vi "mod_query.vi"(5 "connection reference":T3) -> ()   [LabVIEW 2018]
uses:
  <vilib>/addons/database/Connection.llb/Conn ObjectReference.ctl
  <vilib>/addons/database/Connection.llb/Conn Execute.vi
  <vilib>/addons/database/Recordset.llb/Rec Fetch Recordset Data (R).vi
  <vilib>/addons/database/_DB Variant To Data/Database Variant To Data.xnode
  <vilib>/addons/database/NI_Database_API.lvlib
panel:
  in  "清除指示灯 2":bool
  in  "查询学生":bool
  in  "学生信息输入框":T1
  out "数值":dbl
  in  "信息框":i32(listbox)
  in  "查询宿舍所住人信息":bool
  in  "清除指示灯":bool
  in  "查询按钮":bool
  in  "信息输入框":T2
  in  "刷新按钮":bool
  in  "已编辑行数组":u32[](array[numeric])
  in  "信息框缓冲备份":string[][](array[string])
  in  "error in (no error)":errorcluster
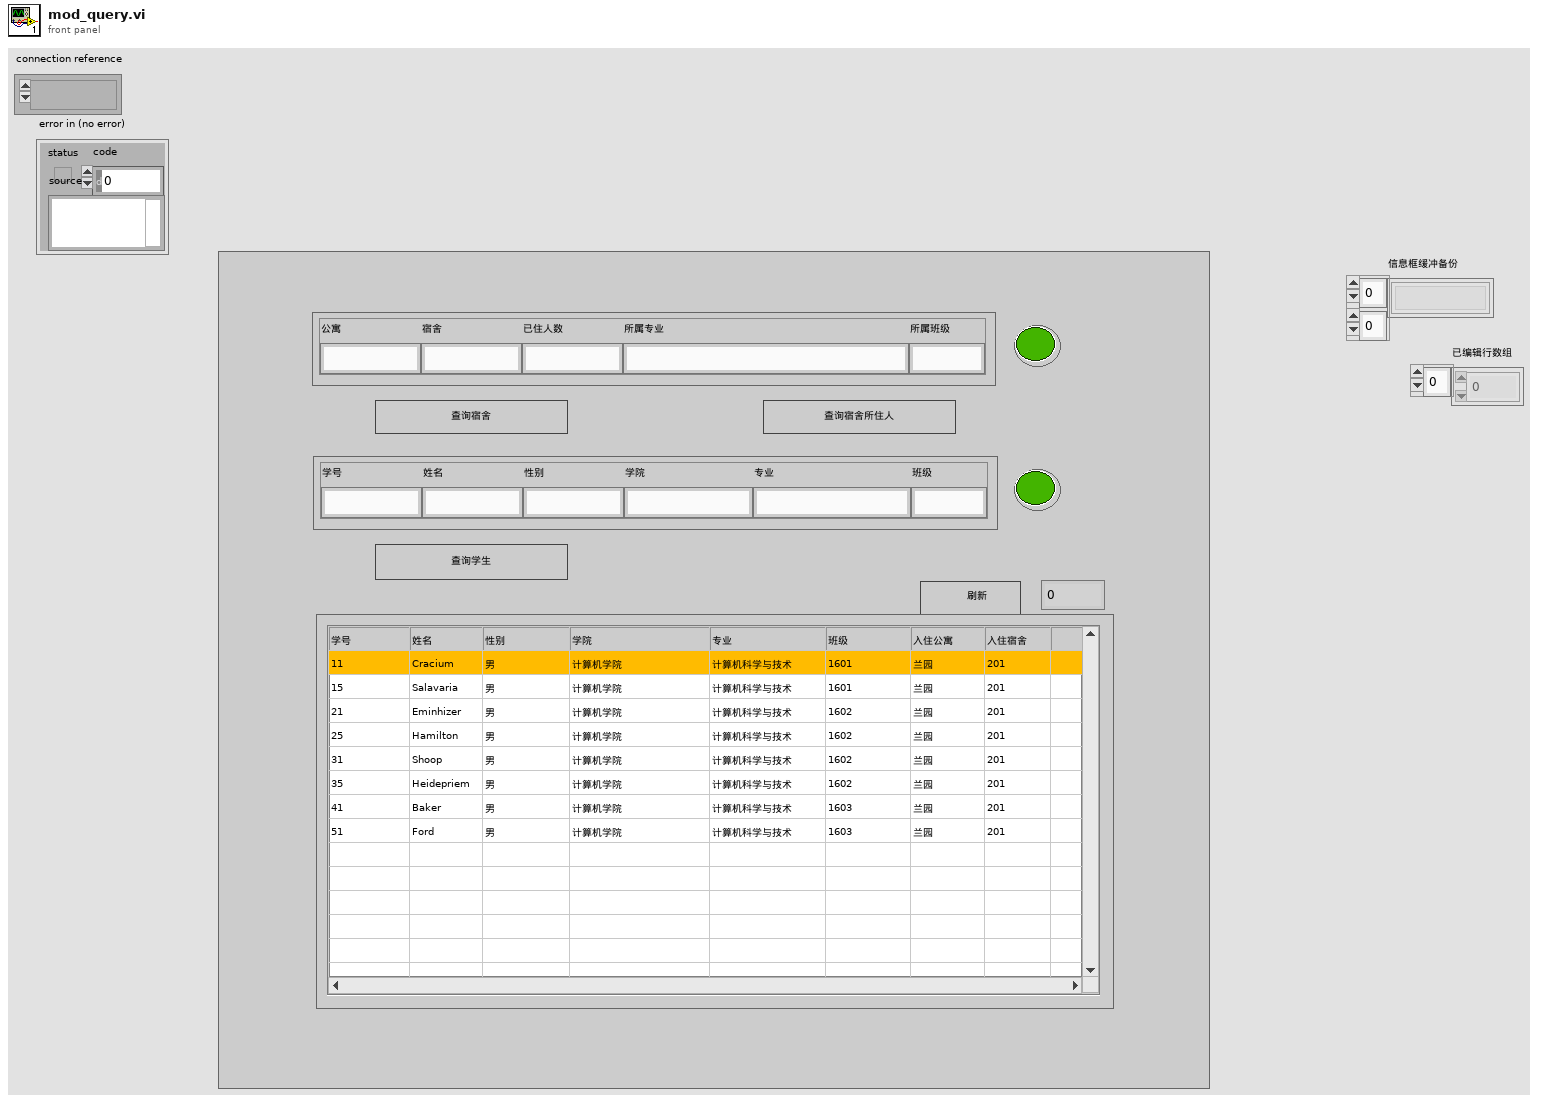
[diagram p1: front panel]
types:
  T1 = cluster{"学号":string, "姓名":string, "性别":string, "学院":string, "专业":string, "班级":string}
  T2 = cluster{"公寓":string, "宿舍":string, "已住人数":string, "所属专业":string, "所属班级":string}
  T3 = typedef "NI_Database_API.lvlib/Conn ObjectReference.ctl" = refnum<k1>
  T4 = cluster{string, string, string, string, string, string, string, string}
  T5 = cluster{string, string, string, string, string, string}
  T6 = typedef "NI_Database_API.lvlib/Rec ObjectReference.ctl" = refnum<k1>
  T7 = cluster{string, string, string, string, string}[]
  T8 = cluster{string, string, string, string, string, string, string, string}[]
  T9 = cluster{string, string, string, string, string, string}[]
  T10 = cluster{"[0]":string, "[1]":string, "[2]":string, "[3]":string, "[4]":string}
  T11 = cluster{"[0]":string, "[1]":string, "[2]":string, "[3]":string, "[4]":string, "[5]":string}
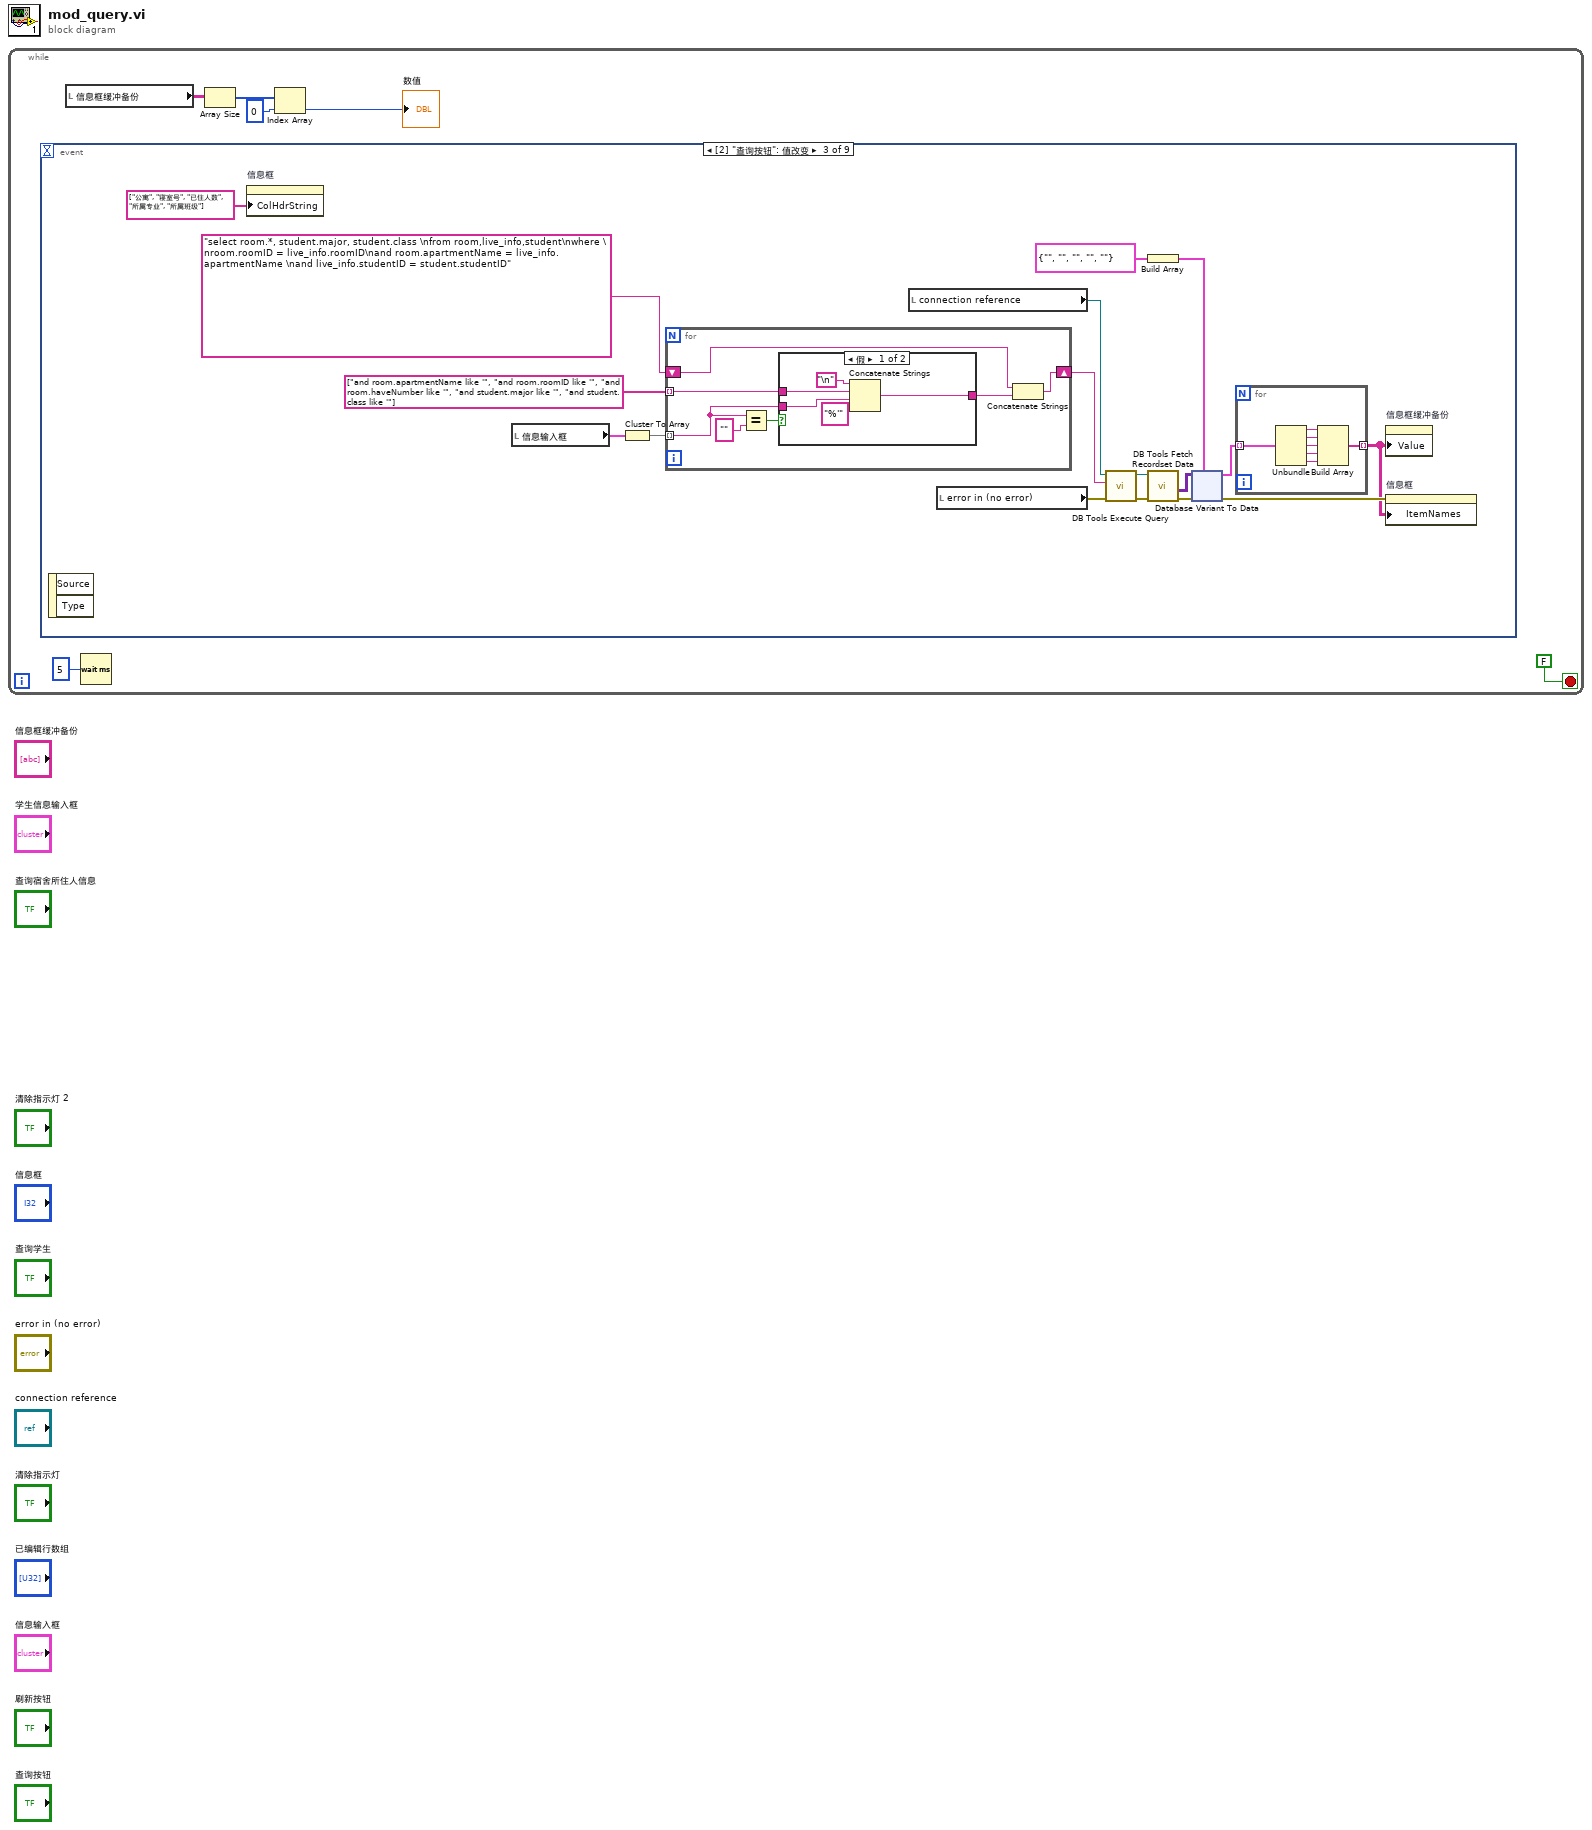
[diagram p0: block diagram]
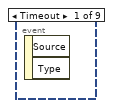
[diagram p2: hidden frame]
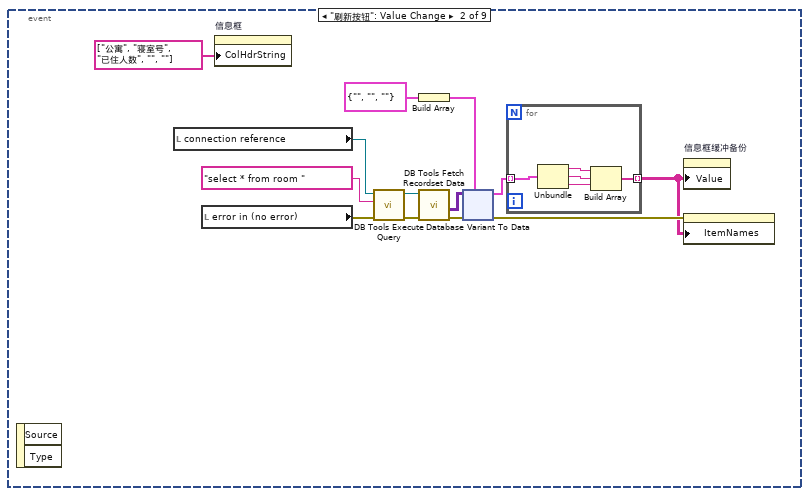
[diagram p3: hidden frame]
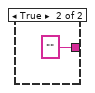
[diagram p4: hidden frame]
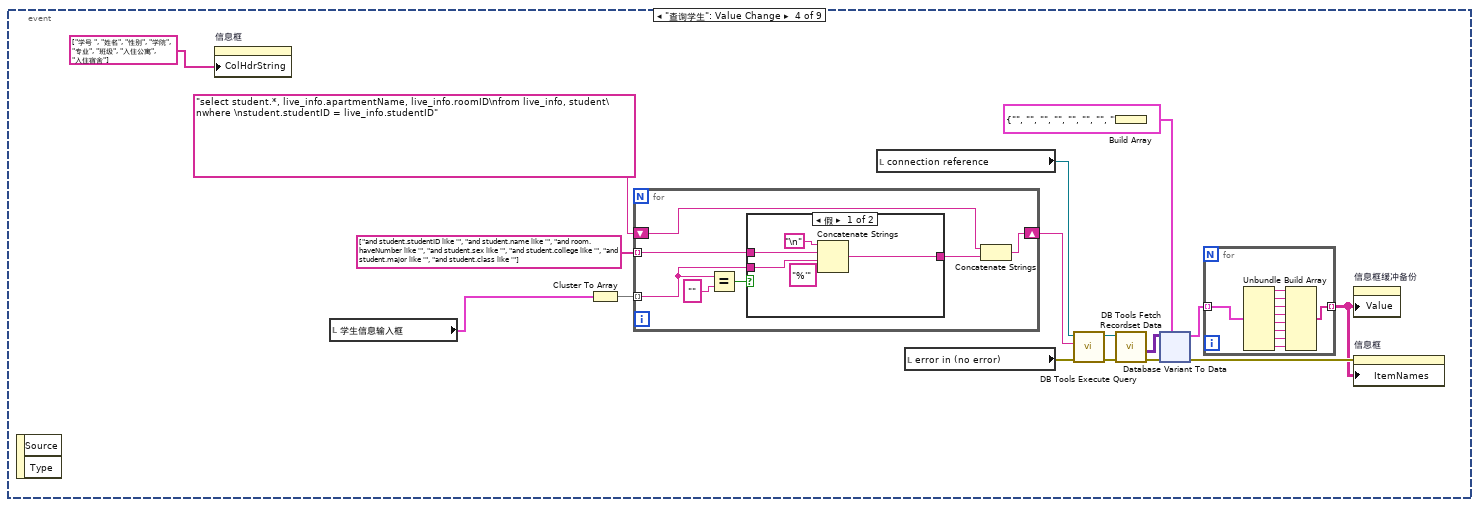
[diagram p5: hidden frame]
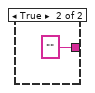
[diagram p6: hidden frame]
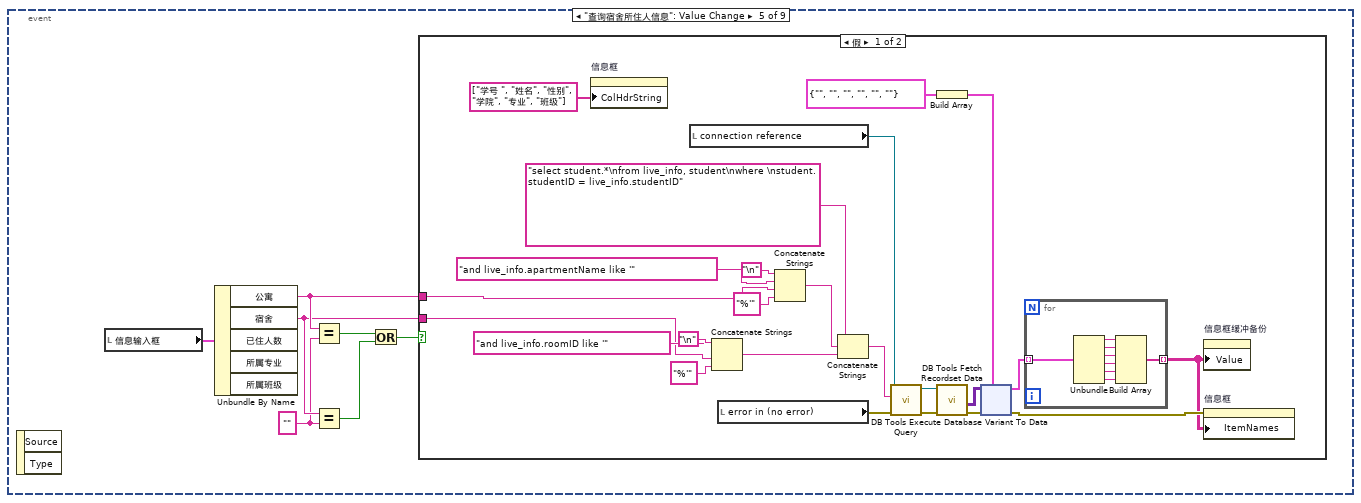
[diagram p7: hidden frame]
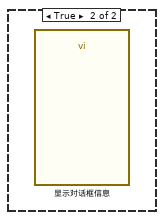
[diagram p8: hidden frame]
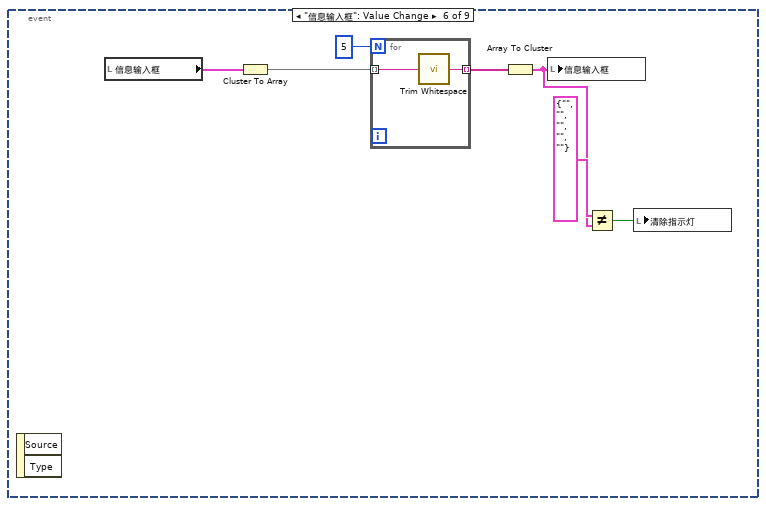
[diagram p9: hidden frame]
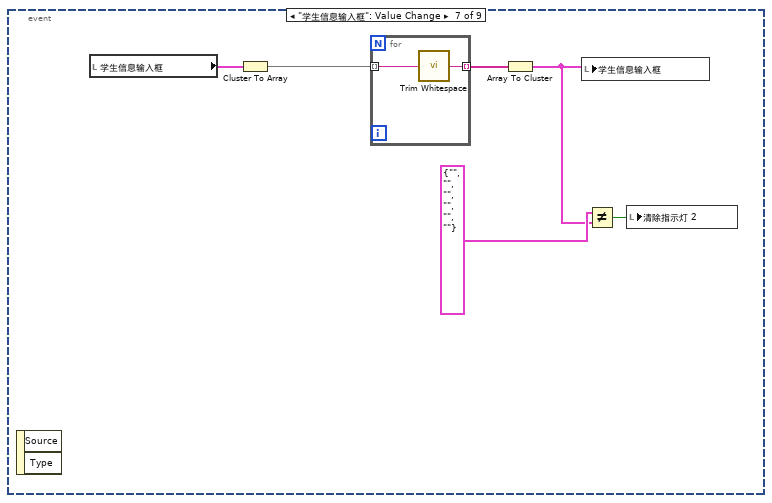
[diagram p10: hidden frame]
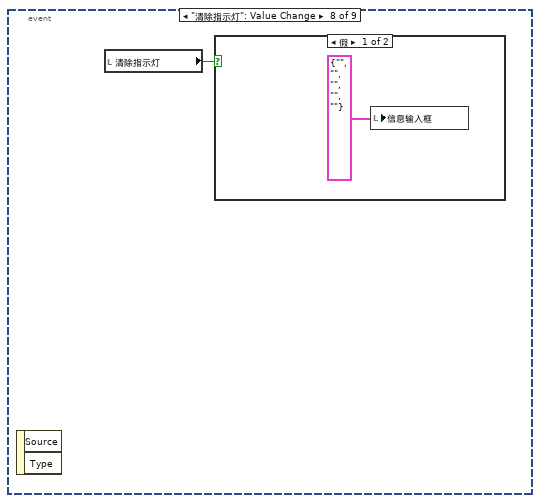
[diagram p11: hidden frame]
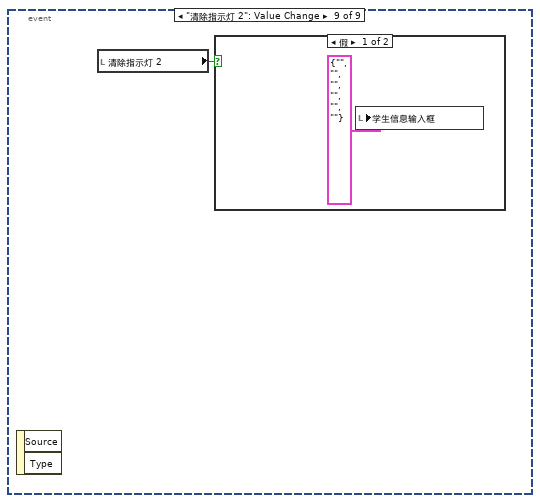
[diagram p13: hidden frame]
diagram:
  n1 = while {
    stop <- FALSE stop-if-true
    n2 = event shown="[2] \"查询按钮\": 值改变" {
      selector: _ -> [_ _ _ _ _ _ _ _ _]
      dyn-events: _ -> [_ _ _ _ _ _ _ _ _]
      timeout: _ -> [_ _ _ _ _ _ _ _ _]
      event Timeout {
        n3 = event-data() -> ()  [unwired: 1 in, 2 out]
      }
      event "刷新按钮": Value Change {
        n4 = event-data() -> ()  [unwired: 1 in, 2 out]
        n5 = local read "connection reference"() -> (w13:T3)
        n6 = local read "error in (no error)"() -> (w12:errorcluster)
        n7 = property on="信息框" class="MCListbox (严格)"("ColHdrString"=string[] ["公寓", "寝室号", "已住人数", "", ""] ("列首字符串[]")) -> ()  [unwired: 2 in, 2 out]
        n8 = call-poly <vilib>:"DB Tools Execute Query.vi"("error in (no error)"=w12, "SQL query"="select * from room ", "connection reference"=w13) -> ("error out"=w15:errorcluster, "recordset reference"=w14:T6)  [unwired: 5 in]
        n9 = Build Array(cluster{string, string, string} {"", "", ""}) -> (w17:cluster{string, string, string}[])
        n10 = call-poly <vilib>:"DB Tools Fetch Recordset Data.vi"("error in (no error)"=w15, "recordset reference"=w14) -> ("error out"=w16:errorcluster, "recordset data"=w11:variant[][])  [unwired: 3 in, 1 out]
        n11 = xnode "Database Variant To Data"("database variant"=w11, "error in (no error)"=w16, "type"=w17) -> ("data"=w18:cluster{string, string, string}[], "error out"=w19:errorcluster)
        n12 = for {
          tunnel: w18 -> [w23] mode=indexing
          tunnel: [w24] -> w8 mode=indexing
          n13 = Unbundle(w23) -> (w21:string, w22:string, w20:string)
          n14 = Build Array(w21, w22, w20) -> (w24:string[])
        }
        n15 = property on="信息框缓冲备份" class="Arr (严格)"("Value"=w8) -> ()  [unwired: 2 in, 2 out]
        n16 = property on="信息框" class="MCListbox (严格)"(error in=w19, "ItemNames"=w8) -> ()  [unwired: 1 in, 2 out]
      }
      event "查询按钮": Value Change {
        n17 = event-data() -> ()  [unwired: 1 in, 2 out]
        n18 = property on="信息框" class="MCListbox (严格)"("ColHdrString"=string[] ["公寓", "寝室号", "已住人数", "所属专业", "所属班级"] ("列首字符串[]")) -> ()  [unwired: 2 in, 2 out]
        n19 = local read "信息输入框"() -> (w134:T2)
        n20 = Cluster To Array(cluster=w134) -> (array=w133:string[])
        n21 = for {
          shift-right: [w147] -> w135
          shift-left: "select room.*, student.major, student.class \nfrom room,live_info,student\nwhere \nroom.roomID = live_info.roomID\nand room.apartmentName = live_info.apartmentName \nand live_info.studentID = student.studentID" -> [w146]
          tunnel: string[] ["and room.apartmentName like '", "and room.roomID like '", "and room.haveNumber like '", "and student.major like '", "and student.class like '"] ("数组") -> [w148] mode=indexing
          tunnel: w133 -> [w149] mode=indexing
          n22 = Equal?(x=w149, y="") -> (x = y?=w151:bool)
          n23 = case shown="假" w151 {
            tunnel: [w152 ""] -> w145
            tunnel: w149 -> [w154 _]
            tunnel: w148 -> [w155 _]
            frame False {
              n24 = Concatenate Strings("\n", w155, w154, "%'") -> (w152:string)
            }
            frame True {
            }
          }
          n25 = Concatenate Strings(w146, w145) -> (w147:string)
        }
        n26 = local read "connection reference"() -> (w144:T3)
        n27 = local read "error in (no error)"() -> (w143:errorcluster)
        n28 = call-poly <vilib>:"DB Tools Execute Query.vi"("error in (no error)"=w143, "SQL query"=w135, "connection reference"=w144) -> ("error out"=w136:errorcluster, "recordset reference"=w137:T6)  [unwired: 5 in]
        n29 = Build Array(cluster{string, string, string, string, string} {"", "", "", "", ""}) -> (w140:T7)
        n30 = call-poly <vilib>:"DB Tools Fetch Recordset Data.vi"("error in (no error)"=w136, "recordset reference"=w137) -> ("error out"=w138:errorcluster, "recordset data"=w139:variant[][])  [unwired: 3 in, 1 out]
        n31 = xnode "Database Variant To Data"("database variant"=w139, "error in (no error)"=w138, "type"=w140) -> ("data"=w141:T7, "error out"=w142:errorcluster)
        n32 = for {
          tunnel: w141 -> [w163] mode=indexing
          tunnel: [w164] -> w128 mode=indexing
          n33 = Unbundle(w163) -> (w162:string, w161:string, w160:string, w159:string, w158:string)
          n34 = Build Array(w162, w161, w160, w159, w158) -> (w164:string[])
        }
        n35 = property on="信息框缓冲备份" class="Arr (严格)"("Value"=w128) -> ()  [unwired: 2 in, 2 out]
        n36 = property on="信息框" class="MCListbox (严格)"(error in=w142, "ItemNames"=w128) -> ()  [unwired: 1 in, 2 out]
      }
      event "查询学生": Value Change {
        n37 = event-data() -> ()  [unwired: 1 in, 2 out]
        n38 = property on="信息框" class="MCListbox (严格)"("ColHdrString"=string[] ["学号 ", "姓名", "性别", "学院", "专业", "班级", "入住公寓", "入住宿舍"] ("列首字符串[]")) -> ()  [unwired: 2 in, 2 out]
        n39 = local read "学生信息输入框"() -> (w330:T1)
        n40 = Cluster To Array(cluster=w330) -> (array=w336:string[])
        n41 = for {
          shift-right: [w349] -> w337
          shift-left: "select student.*, live_info.apartmentName, live_info.roomID\nfrom live_info, student\nwhere \nstudent.studentID = live_info.studentID" -> [w348]
          tunnel: string[] ["and student.studentID like '", "and student.name like '", "and room.haveNumber like '", "and student.sex like '", "and student.college like '", "and student.major like '", "and student.class like '"] ("数组") -> [w350] mode=indexing
          tunnel: w336 -> [w351] mode=indexing
          n42 = Equal?(x=w351, y="") -> (x = y?=w353:bool)
          n43 = case shown="假" w353 {
            tunnel: [w354 ""] -> w347
            tunnel: w351 -> [w356 _]
            tunnel: w350 -> [w357 _]
            frame False {
              n44 = Concatenate Strings("\n", w357, w356, "%'") -> (w354:string)
            }
            frame True {
            }
          }
          n45 = Concatenate Strings(w348, w347) -> (w349:string)
        }
        n46 = local read "connection reference"() -> (w346:T3)
        n47 = local read "error in (no error)"() -> (w345:errorcluster)
        n48 = call-poly <vilib>:"DB Tools Execute Query.vi"("error in (no error)"=w345, "SQL query"=w337, "connection reference"=w346) -> ("error out"=w338:errorcluster, "recordset reference"=w339:T6)  [unwired: 5 in]
        n49 = Build Array(T4 {"", "", "", "", "", "", "", ""}) -> (w342:T8)
        n50 = call-poly <vilib>:"DB Tools Fetch Recordset Data.vi"("error in (no error)"=w338, "recordset reference"=w339) -> ("error out"=w340:errorcluster, "recordset data"=w341:variant[][])  [unwired: 3 in, 1 out]
        n51 = xnode "Database Variant To Data"("database variant"=w341, "error in (no error)"=w340, "type"=w342) -> ("data"=w343:T8, "error out"=w344:errorcluster)
        n52 = for {
          tunnel: w343 -> [w368] mode=indexing
          tunnel: [w369] -> w332 mode=indexing
          n53 = Unbundle(w368) -> (w367:string, w366:string, w365:string, w364:string, w363:string, w360:string, w361:string, w362:string)
          n54 = Build Array(w367, w366, w365, w364, w363, w360, w361, w362) -> (w369:string[])
        }
        n55 = property on="信息框缓冲备份" class="Arr (严格)"("Value"=w332) -> ()  [unwired: 2 in, 2 out]
        n56 = property on="信息框" class="MCListbox (严格)"(error in=w344, "ItemNames"=w332) -> ()  [unwired: 1 in, 2 out]
      }
      event "查询宿舍所住人信息": Value Change {
        w628 = ""
        n57 = event-data() -> ()  [unwired: 1 in, 2 out]
        n58 = local read "信息输入框"() -> (w634:T2)
        n59 = Unbundle By Name(w634) -> ("公寓"=w633:string, "宿舍"=w629:string)  [unwired: 3 out]
        n60 = Equal?(x=w633, y=w628) -> (x = y?=w631:bool)
        n61 = Equal?(x=w629, y=w628) -> (x = y?=w630:bool)
        n62 = Or(x=w631, y=w630) -> (x .or. y?=w632:bool)
        n63 = case shown="假" w632 {
          tunnel: w633 -> [w643 _]
          tunnel: w629 -> [w635 _]
          frame False {
            n64 = property on="信息框" class="MCListbox (严格)"("ColHdrString"=string[] ["学号 ", "姓名", "性别", "学院", "专业", "班级"] ("列首字符串[]")) -> ()  [unwired: 2 in, 2 out]
            n65 = local read "connection reference"() -> (w658:T3)
            n66 = Concatenate Strings("\n", "and live_info.roomID like '" ("字符串"), w635, "%'" ("字符串")) -> (w639:string)
            n67 = local read "error in (no error)"() -> (w657:errorcluster)
            n68 = Concatenate Strings("\n", "and live_info.apartmentName like '" ("字符串"), w643, "%'" ("字符串")) -> (w640:string)
            n69 = Concatenate Strings("select student.*\nfrom live_info, student\nwhere \nstudent.studentID = live_info.studentID", w640, w639) -> (w646:string)
            n70 = call-poly <vilib>:"DB Tools Execute Query.vi"("error in (no error)"=w657, "SQL query"=w646, "connection reference"=w658) -> ("error out"=w650:errorcluster, "recordset reference"=w651:T6)  [unwired: 5 in]
            n71 = Build Array(T5 {"", "", "", "", "", ""}) -> (w654:T9)
            n72 = call-poly <vilib>:"DB Tools Fetch Recordset Data.vi"("error in (no error)"=w650, "recordset reference"=w651) -> ("error out"=w652:errorcluster, "recordset data"=w653:variant[][])  [unwired: 3 in, 1 out]
            n73 = xnode "Database Variant To Data"("database variant"=w653, "error in (no error)"=w652, "type"=w654) -> ("data"=w655:T9, "error out"=w656:errorcluster)
            n74 = for {
              tunnel: w655 -> [w665] mode=indexing
              tunnel: [w666] -> w648 mode=indexing
              n75 = Unbundle(w665) -> (w664:string, w663:string, w662:string, w661:string, w660:string, w659:string)
              n76 = Build Array(w664, w663, w662, w661, w660, w659) -> (w666:string[])
            }
            n77 = property on="信息框缓冲备份" class="Arr (严格)"("Value"=w648) -> ()  [unwired: 2 in, 2 out]
            n78 = property on="信息框" class="MCListbox (严格)"(error in=w656, "ItemNames"=w648) -> ()  [unwired: 1 in, 2 out]
          }
          frame True {
            n79 = call "显示对话框信息"() -> ()  [unwired: 10 in, 2 out]
          }
        }
      }
      event "信息输入框": Value Change {
        n80 = event-data() -> ()  [unwired: 1 in, 2 out]
        n81 = local read "信息输入框"() -> (w868:T2)
        n82 = Cluster To Array(cluster=w868) -> (array=w867:string[])
        n83 = for {
          N: 5 -> [_]
          tunnel: w867 -> [w871] mode=indexing
          tunnel: [w870] -> w869 mode=indexing
          n84 = call <vilib>:"Trim Whitespace.vi"("string"=w871) -> ("trimmed string"=w870:string)  [unwired: 1 in]
        }
        n85 = Array To Cluster(array=w869) -> (cluster=w863:T10)
        n86 = local write "信息输入框"(w863) -> ()
        n87 = Not Equal?(x=cluster{string, string, string, string, string} {"", "", "", "", ""}, y=w863) -> (x != y?=w865:bool)
        n88 = local write "清除指示灯"(w865) -> ()
      }
      event "学生信息输入框": Value Change {
        n89 = event-data() -> ()  [unwired: 1 in, 2 out]
        n90 = local read "学生信息输入框"() -> (w876:T1)
        n91 = Cluster To Array(cluster=w876) -> (array=w875:string[])
        n92 = for {
          tunnel: w875 -> [w879] mode=indexing
          tunnel: [w878] -> w877 mode=indexing
          n93 = call <vilib>:"Trim Whitespace.vi"("string"=w879) -> ("trimmed string"=w878:string)  [unwired: 1 in]
        }
        n94 = Array To Cluster(array=w877) -> (cluster=w872:T11)
        n95 = local write "学生信息输入框"(w872) -> ()
        n96 = Not Equal?(x=T5 {"", "", "", "", "", ""}, y=w872) -> (x != y?=w874:bool)
        n97 = local write "清除指示灯 2"(w874) -> ()
      }
      event "清除指示灯": Value Change {
        n98 = event-data() -> ()  [unwired: 1 in, 2 out]
        n99 = local read "清除指示灯"() -> (w880:bool)
        n100 = case shown="假" w880 {
          frame False {
            n101 = local write "信息输入框"(cluster{string, string, string, string, string} {"", "", "", "", ""}) -> ()
          }
          frame True {
          }
        }
      }
      event "清除指示灯 2": Value Change {
        n102 = event-data() -> ()  [unwired: 1 in, 2 out]
        n103 = local read "清除指示灯 2"() -> (w882:bool)
        n104 = case shown="假" w882 {
          frame False {
            n105 = local write "学生信息输入框"(T5 {"", "", "", "", "", ""}) -> ()
          }
          frame True {
          }
        }
      }
    }
    n106 = local read "信息框缓冲备份"() -> (w4:string[][])
    n107 = Wait (ms)(milliseconds to wait=u32 5 ("等待时间（毫秒）")) -> ()  [unwired: 1 out]
    n108 = Array Size(array=w4) -> (size(s)=w2:i32[])
    n109 = Index Array(array=w2, index=0 ("索引")) -> (element=→"数值":i32)
  }
